vi "check_ROI_isEmpty.vi"(1 "ROI":T1) -> (0 "empty?":bool)   [LabVIEW 2015]
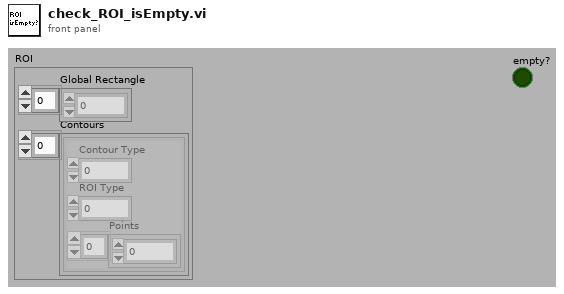
[diagram p1: front panel]
types:
  T1 = cluster{"Global Rectangle":i32[], "Contours":cluster{"Contour Type":u32, "ROI Type":u32, "Points":i32[]}[]}
  T2 = cluster{"Contour Type":u32, "ROI Type":u32, "Points":i32[]}[]
  T3 = cluster{"Contour Type":u32, "ROI Type":u32, "Points":i32[]}
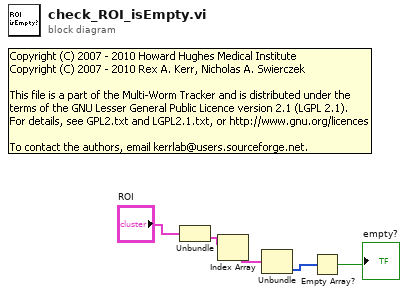
[diagram p0: block diagram]
diagram:
  n1 = Unbundle("ROI") -> ("Contours"=w5:T2)  [unwired: 1 out]
  n2 = Index Array(array=w5) -> (element=w4:T3)  [unwired: 1 in]
  n3 = Unbundle(w4) -> ("Points"=w2:i32[])  [unwired: 2 out]
  n4 = Empty Array?(array=w2) -> (empty?=→"empty?":bool)
